vi "timeout.vi"(8 "error in (no error)":errorcluster, 11 "SpectrographHeartbeat in":refnum<class "SpectrographHeartbeat.lvclass">) -> (0 "error out":errorcluster, 2 "timeout?":bool, 3 "SpectrographHeartbeat out":refnum<class "SpectrographHeartbeat.lvclass">)   [LabVIEW 2016, in "SpectrographHeartbeat.lvclass"]
uses:
  SpectrographHeartbeat.lvclass
  SpectrographHeartbeat.lvclass/SpectrographHeartbeat.ctl
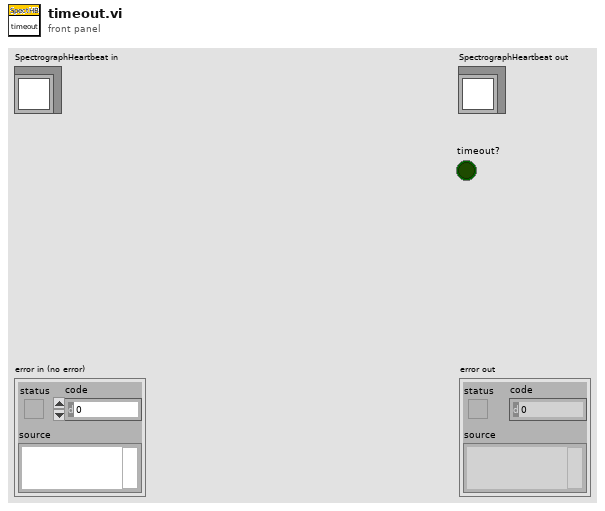
[diagram p1: front panel]
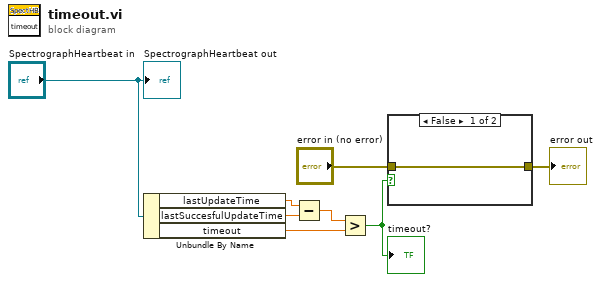
[diagram p0: block diagram]
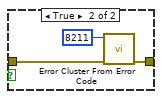
[diagram p2: hidden frame]
diagram:
  n1 = Unbundle By Name("SpectrographHeartbeat in") -> ("lastUpdateTime"=w6:dbl, "lastSuccesfulUpdateTime"=w4:dbl, "timeout"=w5:dbl)
  n2 = Subtract(x=w6, y=w4) -> (x-y=w7:dbl)
  n3 = Greater?(x=w7, y=w5) -> (0:w3:bool)
  "timeout?" <- w3
  n4 = case shown="False" w3 {
    tunnel: "error in (no error)" -> [w9 w12]
    tunnel: [w9 w11] -> w1
    frame False {
    }
    frame True {
      n5 = call <vilib>:"Error Cluster From Error Code.vi"("error in (no error)"=w12, "error code (0)"=8211) -> ("error out"=w11:errorcluster)  [unwired: 7 in]
    }
  }
  "error out" <- w1
  "SpectrographHeartbeat out" <- "SpectrographHeartbeat in"
